vi "Create.vi"(8 "error in (no error)":errorcluster, 10 "simple Class in":refnum<class "Simple Class.lvclass">, 11 "ID tag":string) -> (0 "error out":errorcluster, 3 "reference Class out":refnum<class "Reference Class.lvclass">)   [LabVIEW 2023, in "Reference Class.lvclass"]
doc: "Use this VI before any other calls to the reference class. It initializes the single-element queue."
uses:
  Reference Class.lvclass
  SimpleClass/Simple Class.lvclass
  Reference Class.lvclass/Reference Class.ctl
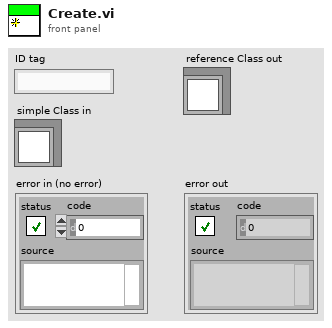
[diagram p1: front panel]
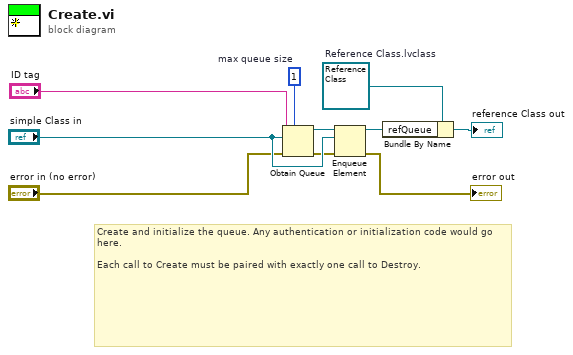
[diagram p0: block diagram]
diagram:
  w3 = refnum<class "Reference Class.lvclass"> refnum  # Reference Class.lvclass
  w5 = 1  # max queue size
  # "Create and initialize the queue. Any authentication or initialization code would go here.\n\nEach call to Create must be paired with exactly one call to Destroy."
  n1 = Obtain Queue(max queue size (-1, unlimited)=w5, name (unnamed)="ID tag", element data type="simple Class in", error in (no error)="error in (no error)") -> (queue out=w8:refnum<queue>, error out=w7:errorcluster)  [unwired: 1 in, 1 out]
  n2 = Enqueue Element(queue=w8, element="simple Class in", error in (no error)=w7) -> (queue out=w2:refnum<queue>, error out=→"error out":errorcluster)  [unwired: 1 in, 1 out]
  n3 = Bundle By Name(cluster=w3, "refQueue"=w2) -> (→"reference Class out":refnum<class "Reference Class.lvclass">)
